vi "ryTimerEx Queue Repeat.vi"() -> ()   [LabVIEW 2020]
uses:
  3122cb75-6530-49f8-9864-937ee694b227.vi
  Lib/ryTimer.lvclass
panel:
  out "Delta Ticks (ms)":i32
  out "Counter":u32
  out "Error":errorcluster
  in  "Exit":bool
  # "Repeats the \"MSG1\"\nevery second."
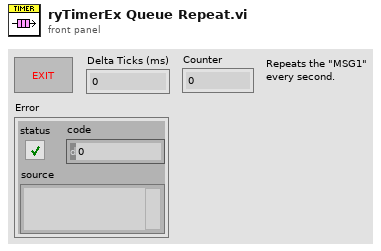
[diagram p1: front panel]
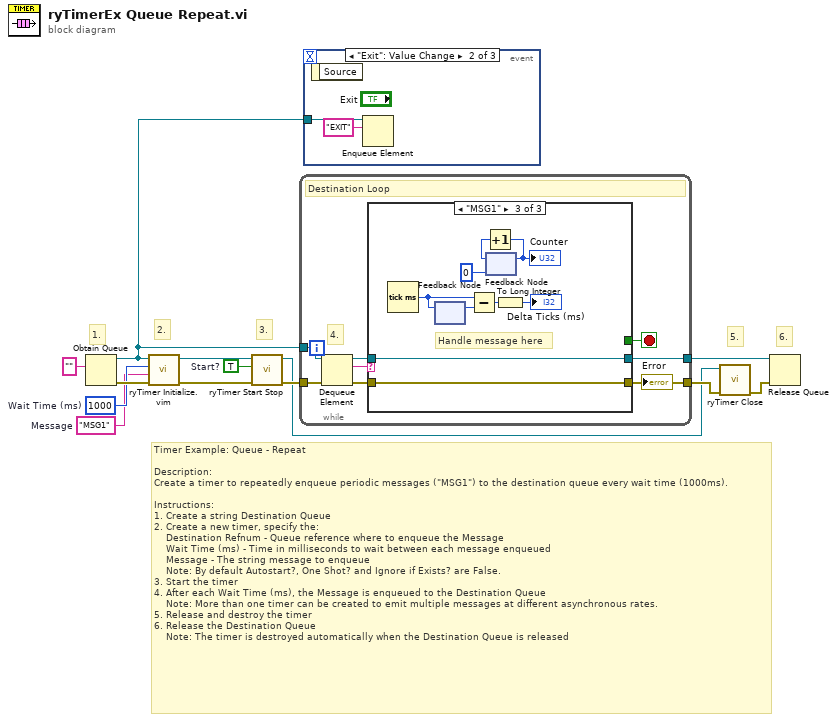
[diagram p0: block diagram]
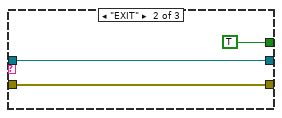
[diagram p3: hidden frame]
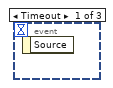
[diagram p4: hidden frame]
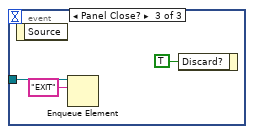
[diagram p5: hidden frame]
diagram:
  w5 = TRUE  # Start?
  w10 = "MSG1"  # Message
  w11 = u32 1000  # Wait Time (ms)
  # "6."
  # "3."
  # "Timer Example: Queue - Repeat\n\nDescription:\nCreate a timer to repeatedly enqueue periodic messages (\"MSG1\") to the destination queue every wait time (1000ms).\n\nInstructions:\n1. Create a string Destination Queue\n2. Create a new timer, specify the:\n    Destination Refnum - Queue reference where to enqueue the Message\n    Wait Time (ms) - Time in milliseconds to wait between each message enqueued\n    Message - The string message to enqueue\n    Note: By default Autostart?, One Shot? and Ignore if Exists? are False.\n3. Start the timer\n4. After each Wait Time (ms), the Message is enqueued to the Destination Queue\n    Note: More than one timer can be created to emit multiple messages at different asynchronous rates.\n5. Release and destroy the timer\n6. Release the Destination Queue\n    Note: The timer is destroyed automatically when the Destination Queue is released"
  # "5."
  # "2."
  # "1."
  n1 = Obtain Queue(element data type="") -> (queue out=w4:refnum<queue>, error out=w12:errorcluster)  [unwired: 4 in, 1 out]
  n2 = call "ryTimer Initialize.vim"("error in (no error)"=w12, "Message"=w10, "Wait Time (ms)"=w11, "Destination Refnum [Q,UE,Any]"=w4) -> ("error out"=w7:errorcluster, "Timer out"=w8:refnum<class "ryTimer.lvclass">)  [unwired: 6 in]
  n3 = call "ryTimer Start Stop.vi"("error in (no error)"=w7, "Start? (F=Stop)"=w5, "Timer in"=w8) -> ("error out"=w6:errorcluster, "Timer out"=w1:refnum<class "ryTimer.lvclass">)  [unwired: 7 in]
  n4 = while {
    tunnel: w4 -> [w21]
    tunnel: [w19] -> w9
    tunnel: w6 -> [w17]
    tunnel: [w14] -> w3
    stop <- w15 stop-if-true
    # "4."
    # "Destination Loop"
    n5 = Dequeue Element(queue=w21, error in (no error)=w17) -> (queue out=w18:refnum<queue>, element=w20:string, error out=w16:errorcluster)  [unwired: 1 in, 1 out]
    n6 = case shown="\"MSG1\"" w20 {
      tunnel: [w23 w26 w35] -> w19
      tunnel: w18 -> [w23 w26 w35]
      tunnel: [w22 w25 w34] -> w14
      tunnel: w16 -> [w22 w25 w34]
      tunnel: [_ TRUE _] -> w15
      frame Default {
      }
      frame "EXIT" {
      }
      frame "MSG1" {
        # "Handle message here"
        n7 = Tick Count (ms)() -> (millisecond timer value=w30:u32)
        n8 = feedback #1() -> (w29:u32)  [unwired: 1 in]
        n9 = feedback-in #1(w30) -> ()
        n10 = Subtract(x=w30, y=w29) -> (x-y=w27:u32)
        n11 = feedback #2(u32 0 ("millisecond timer value")) -> (w32:u32)
        n12 = Increment(x=w32) -> (x+1=w31:u32)
        "Counter" <- w31
        n13 = feedback-in #2(w31) -> ()
        n14 = To Long Integer(number=w27) -> (32bit integer=→"Delta Ticks (ms)":i32)
      }
    }
    "Error" <- w14
  }
  n15 = event shown="[1] \"Exit\": Value Change" {
    selector: _ -> [_ _ _]
    dyn-events: _ -> [_ _ _]
    timeout: _ -> [_ _ _]
    tunnel: w4 -> [_ w37 w40]
    event Timeout {
      n16 = event-data() -> ()  [unwired: 1 in, 1 out]
    }
    event "Exit": Value Change {
      n17 = event-data() -> ()  [unwired: 1 in, 1 out]
      n18 = Enqueue Element(queue=w37, element="EXIT") -> ()  [unwired: 2 in, 3 out]
    }
    event Panel Close? {
      n19 = event-data() -> ()  [unwired: 1 in, 1 out]
      n20 = Enqueue Element(queue=w40, element="EXIT") -> ()  [unwired: 2 in, 3 out]
      n21 = event-data("Discard?"=TRUE) -> ()  [unwired: 1 in, 1 out]
    }
  }
  n22 = call "ryTimer Close.vi"("error in (no error)"=w3, "Timer in"=w1) -> ("error out"=w2:errorcluster)  [unwired: 9 in]
  n23 = Release Queue(queue=w9, error in (no error)=w2) -> ()  [unwired: 1 in, 3 out]
